vi "main.vi"() -> ()   [LabVIEW 2022 SP3]
uses:
  <vilib>/Analysis/Matrix/Datatypes/ComplexMatrix.ctl
  <vilib>/Math Plots/3D Math Plots/3D Bar/3D Bar XCtrl/3D Bar.xctl
  <vilib>/Analysis/baseanly.llb/Complex A x B.vi
  <vilib>/Math Plots/3D Math Plots/3D Bar/3D Bar Datatype/Public/Plot Helper (Matrix).vi
  <vilib>/Analysis/NI_AALBase.lvlib
  <vilib>/Math Plots/3D Math Plots/3D Bar/3D Bar Datatype/3D Bar Datatype.lvclass
  <vilib>/Analysis/Matrix/NI_Matrix.lvlib
panel:
  in  "rhoR":cdb[][](array[numeric])
  in  "rhoL":cdb[][](array[numeric])
  in  "rhoD":cdb[][](array[numeric])
  in  "rhoV":cdb[][](array[numeric])
  in  "rhoH":cdb[][](array[numeric])
  in  "Linear tomography of two photons based on PhysRevA.64.052312.\nPlease note the M matrix in appendix of the paper is not correct.":enum32{"Two photons"}(tab)
  out "Re":refnum<class "3D Plot Datatype.lvclass">[](xcontrol)
  in  "OK Button":bool
  out "Density Matrix":T1
  out "Measurements":string[][](array[string])
  in  "Coincidence counts":i32[](array[numeric])
  out "Im":refnum<class "3D Plot Datatype.lvclass">[](xcontrol)
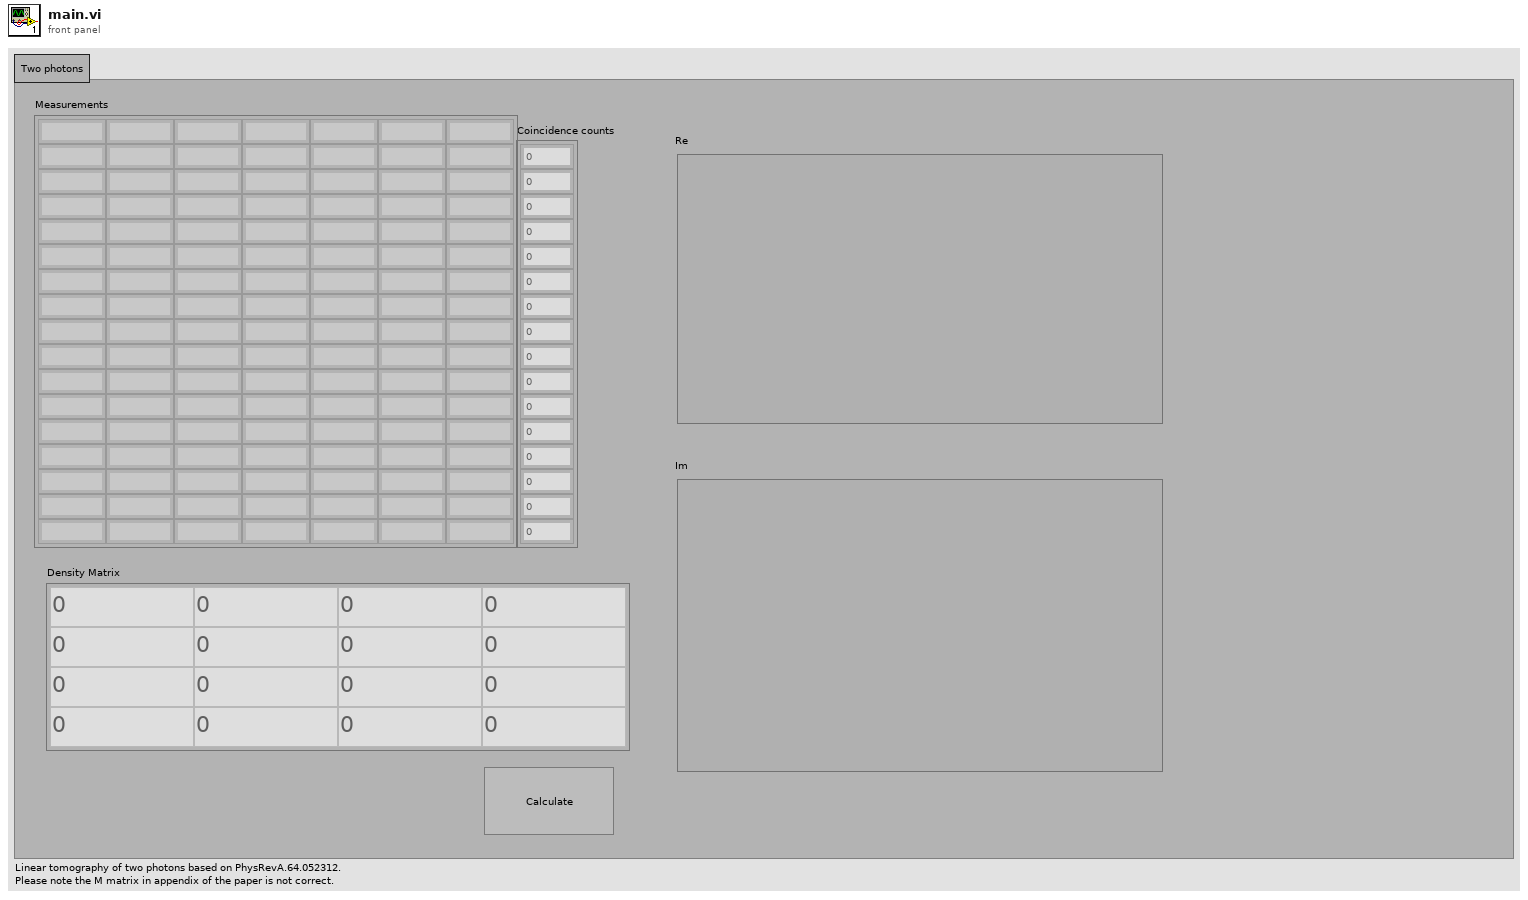
[diagram p1: front panel]
types:
  T1 = typedef "NI_Matrix.lvlib/ComplexMatrix.ctl" = cdb[][]
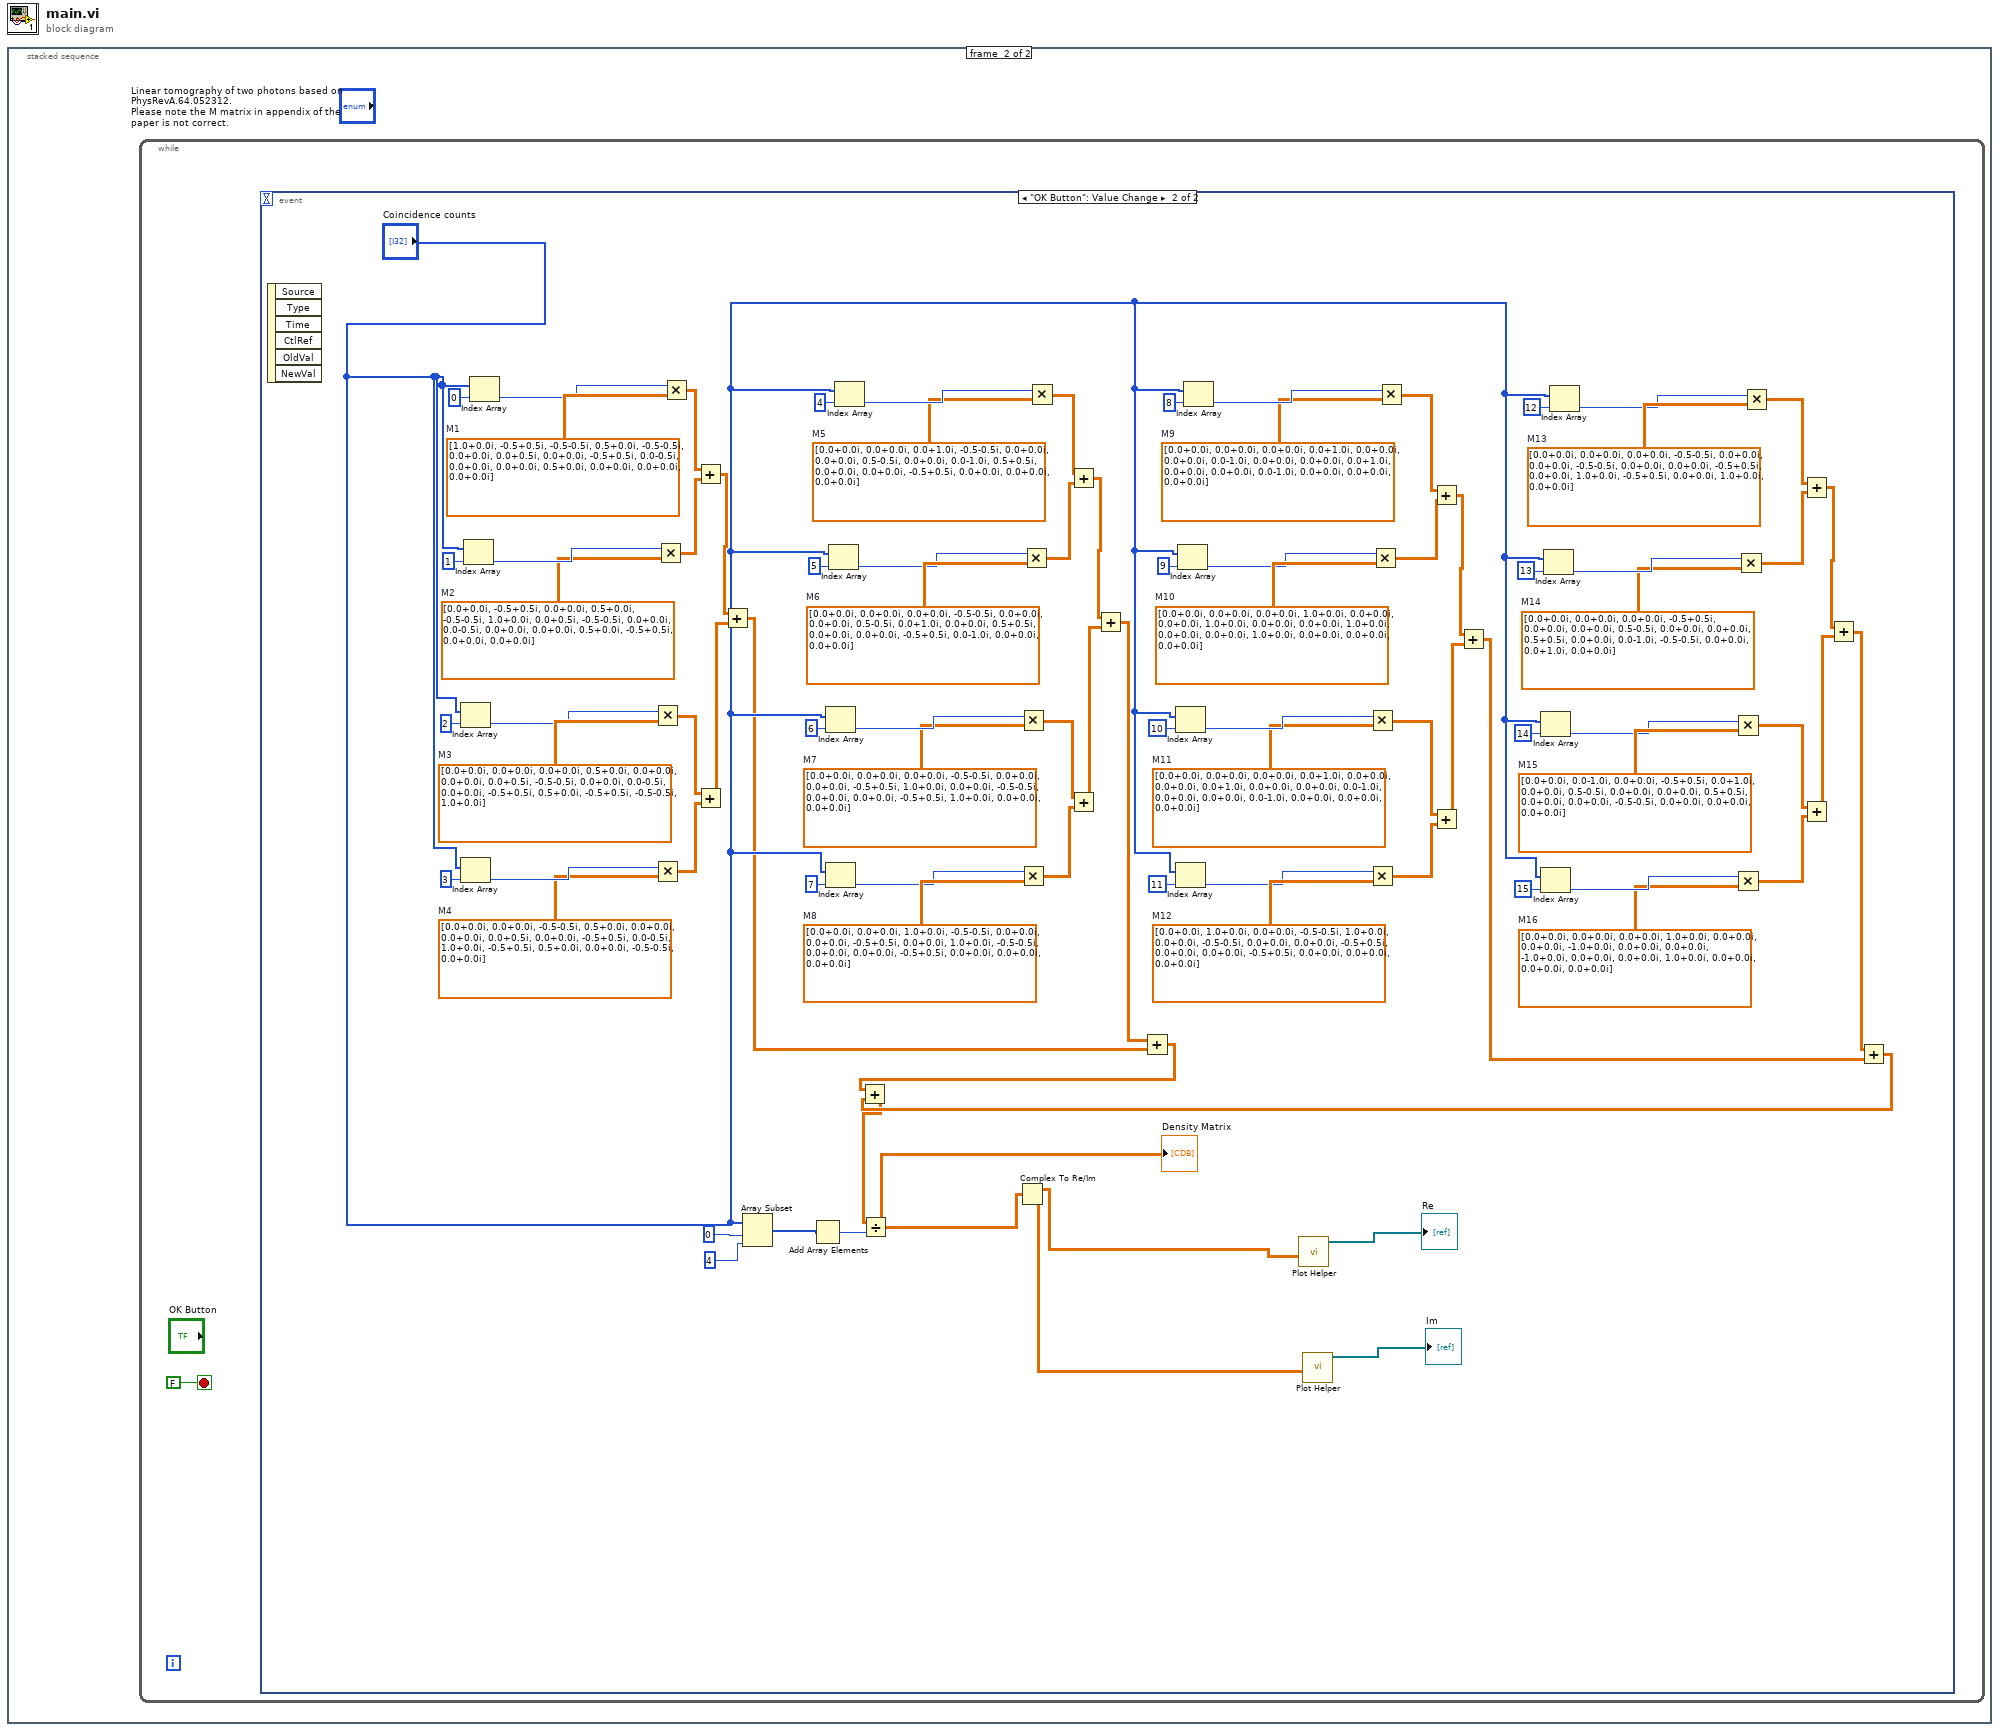
[diagram p0: block diagram]
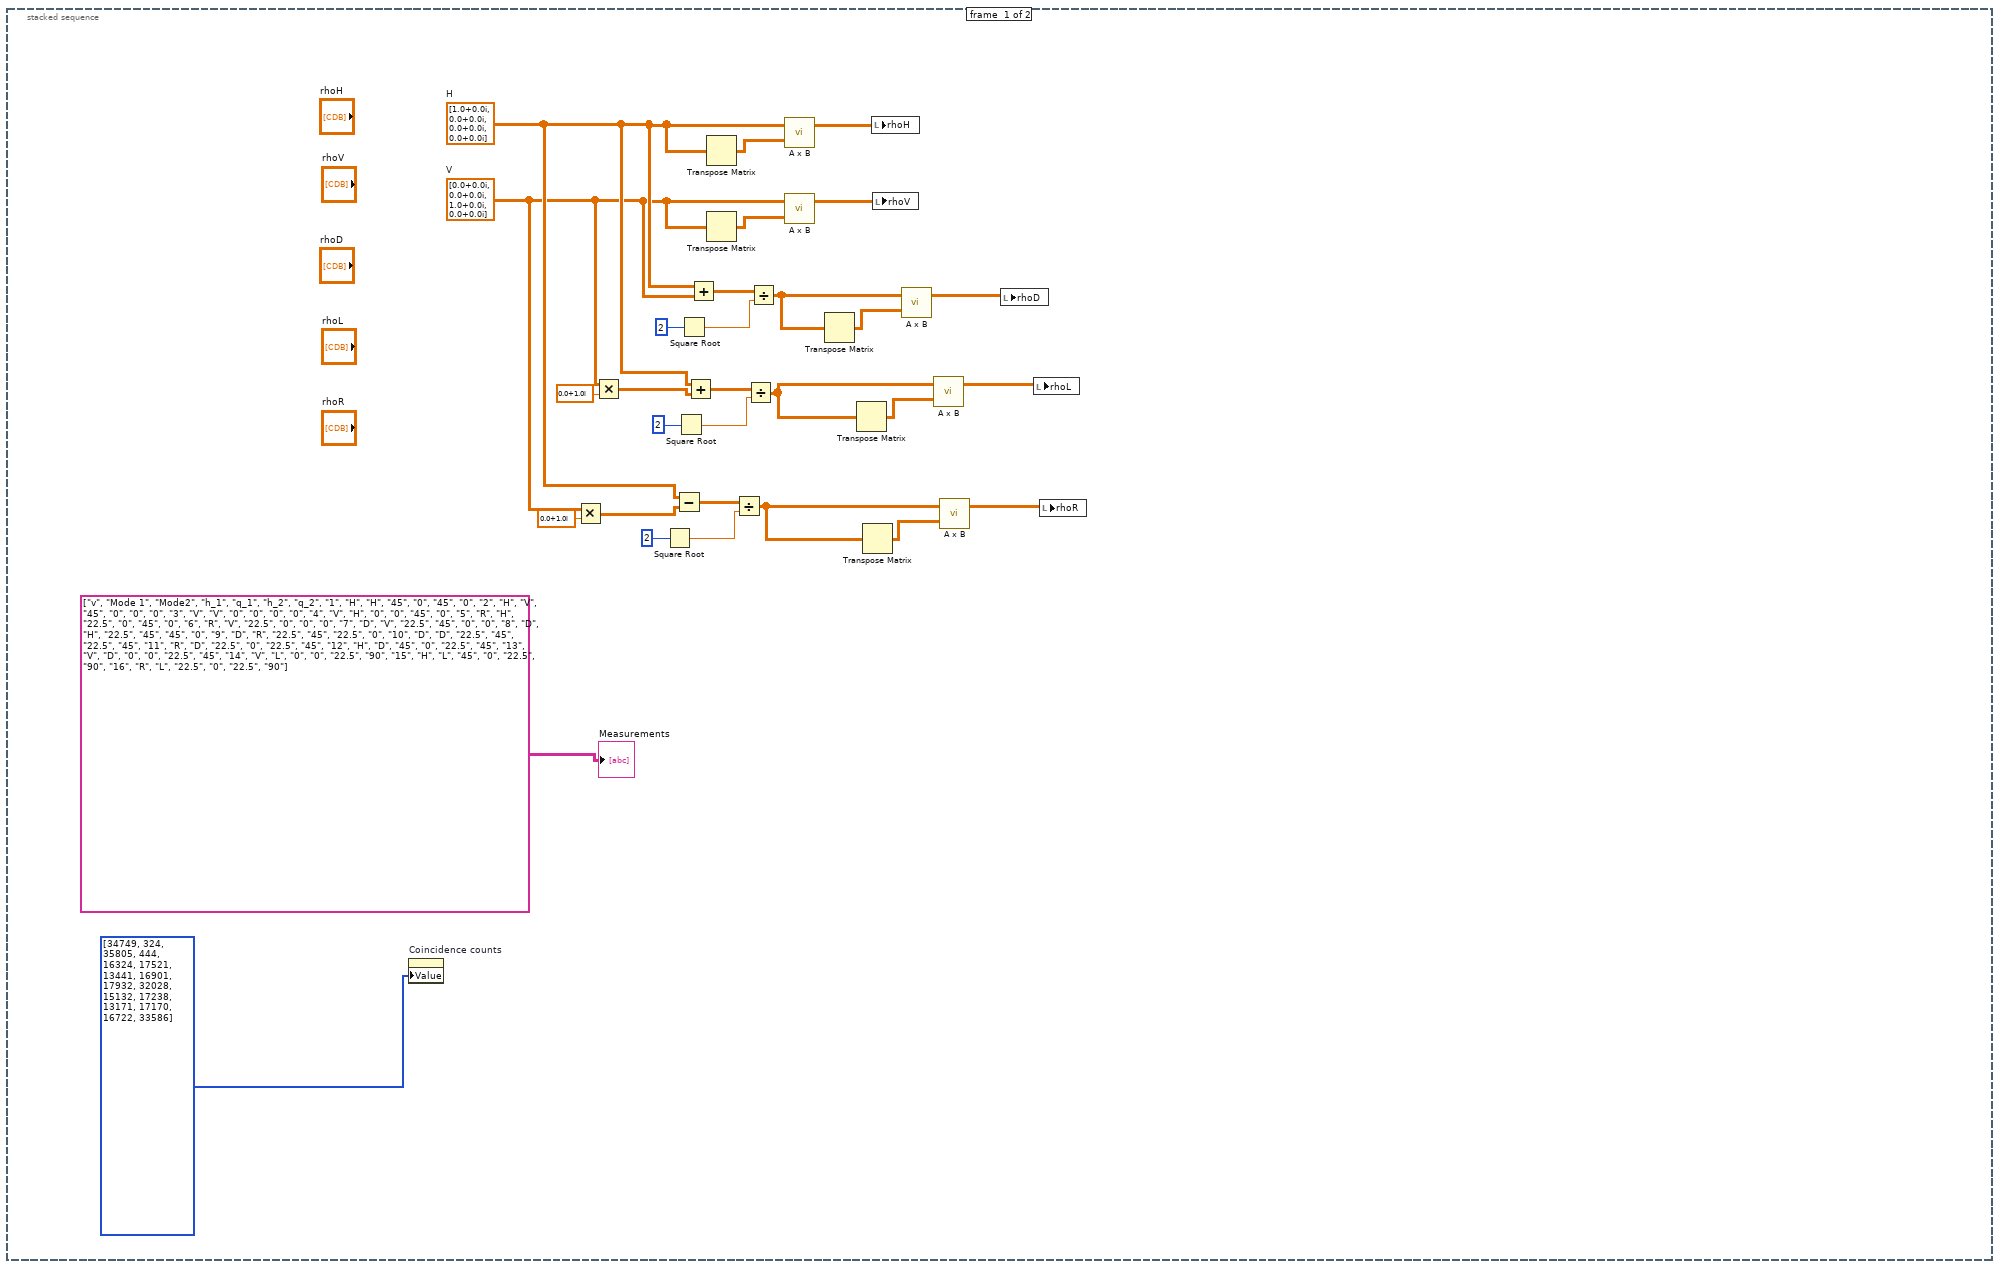
[diagram p2: hidden frame]
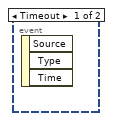
[diagram p3: hidden frame]
diagram:
  n1 = stacked-sequence {
    frame #0 {
      w12 = cdb[][] [[0.0+0.0i, 0.0+0.0i], [1.0+0.0i, 0.0+0.0i]]  # V
      w13 = cdb[][] [[1.0+0.0i, 0.0+0.0i], [0.0+0.0i, 0.0+0.0i]]  # H
      n2 = property on="Coincidence counts" class="Arr (strict)"("Value"=i32[] [34749, 324, 35805, 444, 16324, 17521, 13441, 16901, 17932, 32028, 15132, 17238, 13171, 17170, 16722, 33586] ("Coincidence counts")) -> ()  [unwired: 2 in, 2 out]
      n3 = Multiply(x=w12, y=cdb 0.0+1.0i) -> (x*y=w17:cdb[][])
      n4 = Multiply(x=w12, y=cdb 0.0+1.0i) -> (x*y=w20:cdb[][])
      n5 = Square Root(x=2) -> (sqrt(x)=w14:dbl)
      n6 = Subtract(x=w13, y=w17) -> (x-y=w16:cdb[][])
      n7 = Square Root(x=2) -> (sqrt(x)=w23:dbl)
      n8 = Square Root(x=2) -> (sqrt(x)=w24:dbl)
      n9 = Add(x=w13, y=w20) -> (x+y=w21:cdb[][])
      n10 = Add(x=w13, y=w12) -> (x+y=w26:cdb[][])
      n11 = Transpose Matrix(1:w13) -> (0:w30:cdb[][])
      n12 = Transpose Matrix(1:w12) -> (0:w27:cdb[][])
      n13 = Divide(x=w16, y=w14) -> (x/y=w3:cdb[][])
      n14 = Divide(x=w21, y=w23) -> (x/y=w4:cdb[][])
      n15 = Divide(x=w26, y=w24) -> (x/y=w11:cdb[][])
      n16 = call-poly <vilib>:"A x B.vi"("B"=w30, "A"=w13) -> ("A x B"=w29:T1)  [unwired: 1 out]
      n17 = call-poly <vilib>:"A x B.vi"("B"=w27, "A"=w12) -> ("A x B"=w28:T1)  [unwired: 1 out]
      n18 = Transpose Matrix(1:w11) -> (0:w10:cdb[][])
      n19 = Transpose Matrix(1:w4) -> (0:w7:cdb[][])
      n20 = Transpose Matrix(1:w3) -> (0:w6:cdb[][])
      n21 = local write "rhoH"(w29) -> ()
      n22 = local write "rhoV"(w28) -> ()
      n23 = call-poly <vilib>:"A x B.vi"("B"=w10, "A"=w11) -> ("A x B"=w9:T1)  [unwired: 1 out]
      n24 = call-poly <vilib>:"A x B.vi"("B"=w7, "A"=w4) -> ("A x B"=w8:T1)  [unwired: 1 out]
      n25 = call-poly <vilib>:"A x B.vi"("B"=w6, "A"=w3) -> ("A x B"=w5:T1)  [unwired: 1 out]
      n26 = local write "rhoD"(w9) -> ()
      n27 = local write "rhoL"(w8) -> ()
      n28 = local write "rhoR"(w5) -> ()
      "Measurements" <- string[][] [["v", "Mode 1", "Mode2", "h_1", "q_1", "h_2", "q_2"], ["1", "H", "H", "45", "0", "45", "0"], ["2", "H", "V", "45", "0", "0", "0"], ["3", "V", "V", "0", "0", "0", "0"], ["4", "V", "H", "0", "0", "45", "0"], ["5", "R", "H", "22.5", "0", "45", "0"], ["6", "R", "V", "22.5", "0", "0", "0"], ["7", "D", "V", "22.5", "45", "0", "0"], ["8", "D", "H", "22.5", "45", "45", "0"], ["9", "D", "R", "22.5", "45", "22.5", "0"], ["10", "D", "D", "22.5", "45", "22.5", "45"], ["11", "R", "D", "22.5", "0", "22.5", "45"], ["12", "H", "D", "45", "0", "22.5", "45"], ["13", "V", "D", "0", "0", "22.5", "45"], ["14", "V", "L", "0", "0", "22.5", "90"], ["15", "H", "L", "45", "0", "22.5", "90"], ["16", "R", "L", "22.5", "0", "22.5", "90"]]
    }
    frame #1 {
      n29 = while {
        stop <- FALSE stop-if-true
        n30 = event shown="[1] \"OK Button\": Value Change" {
          selector: _ -> [_ _]
          dyn-events: _ -> [_ _]
          timeout: _ -> [_ _]
          event Timeout {
            n31 = event-data() -> ()  [unwired: 1 in, 3 out]
          }
          event "OK Button": Value Change {
            w82 = cdb[][] [[0.0+0.0i, 0.0+0.0i, 0.0+0.0i, 1.0+0.0i], [0.0+0.0i, 0.0+0.0i, -1.0+0.0i, 0.0+0.0i], [0.0+0.0i, -1.0+0.0i, 0.0+0.0i, 0.0+0.0i], [1.0+0.0i, 0.0+0.0i, 0.0+0.0i, 0.0+0.0i]]  # M16
            w85 = cdb[][] [[0.0+0.0i, 0.0-1.0i, 0.0+0.0i, -0.5+0.5i], [0.0+1.0i, 0.0+0.0i, 0.5-0.5i, 0.0+0.0i], [0.0+0.0i, 0.5+0.5i, 0.0+0.0i, 0.0+0.0i], [-0.5-0.5i, 0.0+0.0i, 0.0+0.0i, 0.0+0.0i]]  # M15
            w88 = cdb[][] [[0.0+0.0i, 0.0+0.0i, 0.0+0.0i, -0.5+0.5i], [0.0+0.0i, 0.0+0.0i, 0.5-0.5i, 0.0+0.0i], [0.0+0.0i, 0.5+0.5i, 0.0+0.0i, 0.0-1.0i], [-0.5-0.5i, 0.0+0.0i, 0.0+1.0i, 0.0+0.0i]]  # M14
            w91 = cdb[][] [[0.0+0.0i, 0.0+0.0i, 0.0+0.0i, -0.5-0.5i], [0.0+0.0i, 0.0+0.0i, -0.5-0.5i, 0.0+0.0i], [0.0+0.0i, -0.5+0.5i, 0.0+0.0i, 1.0+0.0i], [-0.5+0.5i, 0.0+0.0i, 1.0+0.0i, 0.0+0.0i]]  # M13
            w79 = cdb[][] [[0.0+0.0i, 1.0+0.0i, 0.0+0.0i, -0.5-0.5i], [1.0+0.0i, 0.0+0.0i, -0.5-0.5i, 0.0+0.0i], [0.0+0.0i, -0.5+0.5i, 0.0+0.0i, 0.0+0.0i], [-0.5+0.5i, 0.0+0.0i, 0.0+0.0i, 0.0+0.0i]]  # M12
            w76 = cdb[][] [[0.0+0.0i, 0.0+0.0i, 0.0+0.0i, 0.0+1.0i], [0.0+0.0i, 0.0+0.0i, 0.0+1.0i, 0.0+0.0i], [0.0+0.0i, 0.0-1.0i, 0.0+0.0i, 0.0+0.0i], [0.0-1.0i, 0.0+0.0i, 0.0+0.0i, 0.0+0.0i]]  # M11
            w73 = cdb[][] [[0.0+0.0i, 0.0+0.0i, 0.0+0.0i, 1.0+0.0i], [0.0+0.0i, 0.0+0.0i, 1.0+0.0i, 0.0+0.0i], [0.0+0.0i, 1.0+0.0i, 0.0+0.0i, 0.0+0.0i], [1.0+0.0i, 0.0+0.0i, 0.0+0.0i, 0.0+0.0i]]  # M10
            w70 = cdb[][] [[0.0+0.0i, 0.0+0.0i, 0.0+0.0i, 0.0+1.0i], [0.0+0.0i, 0.0+0.0i, 0.0-1.0i, 0.0+0.0i], [0.0+0.0i, 0.0+1.0i, 0.0+0.0i, 0.0+0.0i], [0.0-1.0i, 0.0+0.0i, 0.0+0.0i, 0.0+0.0i]]  # M9
            w103 = cdb[][] [[0.0+0.0i, 0.0+0.0i, 1.0+0.0i, -0.5-0.5i], [0.0+0.0i, 0.0+0.0i, -0.5+0.5i, 0.0+0.0i], [1.0+0.0i, -0.5-0.5i, 0.0+0.0i, 0.0+0.0i], [-0.5+0.5i, 0.0+0.0i, 0.0+0.0i, 0.0+0.0i]]  # M8
            w100 = cdb[][] [[0.0+0.0i, 0.0+0.0i, 0.0+0.0i, -0.5-0.5i], [0.0+0.0i, 0.0+0.0i, -0.5+0.5i, 1.0+0.0i], [0.0+0.0i, -0.5-0.5i, 0.0+0.0i, 0.0+0.0i], [-0.5+0.5i, 1.0+0.0i, 0.0+0.0i, 0.0+0.0i]]  # M7
            w97 = cdb[][] [[0.0+0.0i, 0.0+0.0i, 0.0+0.0i, -0.5-0.5i], [0.0+0.0i, 0.0+0.0i, 0.5-0.5i, 0.0+1.0i], [0.0+0.0i, 0.5+0.5i, 0.0+0.0i, 0.0+0.0i], [-0.5+0.5i, 0.0-1.0i, 0.0+0.0i, 0.0+0.0i]]  # M6
            w94 = cdb[][] [[0.0+0.0i, 0.0+0.0i, 0.0+1.0i, -0.5-0.5i], [0.0+0.0i, 0.0+0.0i, 0.5-0.5i, 0.0+0.0i], [0.0-1.0i, 0.5+0.5i, 0.0+0.0i, 0.0+0.0i], [-0.5+0.5i, 0.0+0.0i, 0.0+0.0i, 0.0+0.0i]]  # M5
            w106 = cdb[][] [[0.0+0.0i, 0.0+0.0i, -0.5-0.5i, 0.5+0.0i], [0.0+0.0i, 0.0+0.0i, 0.0+0.5i, 0.0+0.0i], [-0.5+0.5i, 0.0-0.5i, 1.0+0.0i, -0.5+0.5i], [0.5+0.0i, 0.0+0.0i, -0.5-0.5i, 0.0+0.0i]]  # M4
            w109 = cdb[][] [[0.0+0.0i, 0.0+0.0i, 0.0+0.0i, 0.5+0.0i], [0.0+0.0i, 0.0+0.0i, 0.0+0.5i, -0.5-0.5i], [0.0+0.0i, 0.0-0.5i, 0.0+0.0i, -0.5+0.5i], [0.5+0.0i, -0.5+0.5i, -0.5-0.5i, 1.0+0.0i]]  # M3
            w112 = cdb[][] [[0.0+0.0i, -0.5+0.5i, 0.0+0.0i, 0.5+0.0i], [-0.5-0.5i, 1.0+0.0i, 0.0+0.5i, -0.5-0.5i], [0.0+0.0i, 0.0-0.5i, 0.0+0.0i, 0.0+0.0i], [0.5+0.0i, -0.5+0.5i, 0.0+0.0i, 0.0+0.0i]]  # M2
            w115 = cdb[][] [[1.0+0.0i, -0.5+0.5i, -0.5-0.5i, 0.5+0.0i], [-0.5-0.5i, 0.0+0.0i, 0.0+0.5i, 0.0+0.0i], [-0.5+0.5i, 0.0-0.5i, 0.0+0.0i, 0.0+0.0i], [0.5+0.0i, 0.0+0.0i, 0.0+0.0i, 0.0+0.0i]]  # M1
            n32 = event-data() -> ()  [unwired: 1 in, 6 out]
            n33 = Index Array(array="Coincidence counts", index=2) -> (element=w108:i32)
            n34 = Index Array(array="Coincidence counts", index=3) -> (element=w107:i32)
            n35 = Index Array(array="Coincidence counts", index=1) -> (element=w113:i32)
            n36 = Index Array(array="Coincidence counts", index=0) -> (element=w114:i32)
            n37 = Multiply(x=w108, y=w109) -> (x*y=w64:cdb[][])
            n38 = Multiply(x=w107, y=w106) -> (x*y=w65:cdb[][])
            n39 = Multiply(x=w113, y=w112) -> (x*y=w66:cdb[][])
            n40 = Multiply(x=w114, y=w115) -> (x*y=w67:cdb[][])
            n41 = Add(x=w67, y=w66) -> (x+y=w63:cdb[][])
            n42 = Add(x=w64, y=w65) -> (x+y=w62:cdb[][])
            n43 = Add(x=w63, y=w62) -> (x+y=w42:cdb[][])
            n44 = Array Subset(array="Coincidence counts", index=0, length=4) -> (w117:i32[])
            n45 = Add Array Elements(numeric array=w117) -> (sum=w118:i32)
            n46 = Index Array(array="Coincidence counts", index=6) -> (element=w101:i32)
            n47 = Index Array(array="Coincidence counts", index=7) -> (element=w102:i32)
            n48 = Index Array(array="Coincidence counts", index=5) -> (element=w96:i32)
            n49 = Index Array(array="Coincidence counts", index=4) -> (element=w95:i32)
            n50 = Multiply(x=w101, y=w100) -> (x*y=w53:cdb[][])
            n51 = Multiply(x=w102, y=w103) -> (x*y=w52:cdb[][])
            n52 = Multiply(x=w96, y=w97) -> (x*y=w54:cdb[][])
            n53 = Multiply(x=w95, y=w94) -> (x*y=w55:cdb[][])
            n54 = Add(x=w55, y=w54) -> (x+y=w60:cdb[][])
            n55 = Add(x=w53, y=w52) -> (x+y=w61:cdb[][])
            n56 = Add(x=w60, y=w61) -> (x+y=w43:cdb[][])
            n57 = Add(x=w43, y=w42) -> (x+y=w39:cdb[][])
            n58 = Index Array(array="Coincidence counts", index=10) -> (element=w77:i32)
            n59 = Index Array(array="Coincidence counts", index=11) -> (element=w78:i32)
            n60 = Index Array(array="Coincidence counts", index=9) -> (element=w72:i32)
            n61 = Index Array(array="Coincidence counts", index=8) -> (element=w71:i32)
            n62 = Multiply(x=w77, y=w76) -> (x*y=w49:cdb[][])
            n63 = Multiply(x=w78, y=w79) -> (x*y=w48:cdb[][])
            n64 = Multiply(x=w72, y=w73) -> (x*y=w50:cdb[][])
            n65 = Multiply(x=w71, y=w70) -> (x*y=w51:cdb[][])
            n66 = Add(x=w51, y=w50) -> (x+y=w59:cdb[][])
            n67 = Add(x=w49, y=w48) -> (x+y=w58:cdb[][])
            n68 = Add(x=w59, y=w58) -> (x+y=w40:cdb[][])
            n69 = Index Array(array="Coincidence counts", index=14) -> (element=w84:i32)
            n70 = Index Array(array="Coincidence counts", index=15) -> (element=w83:i32)
            n71 = Index Array(array="Coincidence counts", index=13) -> (element=w89:i32)
            n72 = Index Array(array="Coincidence counts", index=12) -> (element=w90:i32)
            n73 = Multiply(x=w84, y=w85) -> (x*y=w45:cdb[][])
            n74 = Multiply(x=w83, y=w82) -> (x*y=w44:cdb[][])
            n75 = Multiply(x=w89, y=w88) -> (x*y=w46:cdb[][])
            n76 = Multiply(x=w90, y=w91) -> (x*y=w47:cdb[][])
            n77 = Add(x=w47, y=w46) -> (x+y=w56:cdb[][])
            n78 = Add(x=w45, y=w44) -> (x+y=w57:cdb[][])
            n79 = Add(x=w56, y=w57) -> (x+y=w41:cdb[][])
            n80 = Add(x=w41, y=w40) -> (x+y=w38:cdb[][])
            n81 = Add(x=w39, y=w38) -> (x+y=w37:cdb[][])
            n82 = Divide(x=w37, y=w118) -> (x/y=w35:cdb[][])
            "Density Matrix" <- w35
            n83 = Complex To Re/Im(x + iy=w35) -> (x=w34:dbl[][], y=w32:dbl[][])
            n84 = call-poly <vilib>:"Plot Helper.vi"("z matrix"=w34) -> ("3D Plot lvclass Array out"=→"Re":refnum<class "3D Plot Datatype.lvclass">[])  [unwired: 2 in, 8 out]
            n85 = call-poly <vilib>:"Plot Helper.vi"("z matrix"=w32) -> ("3D Plot lvclass Array out"=→"Im":refnum<class "3D Plot Datatype.lvclass">[])  [unwired: 2 in, 8 out]
          }
        }
      }
    }
  }
